vi "Queue_0125.vi"() -> ()   [LabVIEW 2021]
panel:
  out "# elements in queue":i32
  out "Consumer":dbl(graph)
  out "Producer":dbl(graph)
  in  "stop":bool
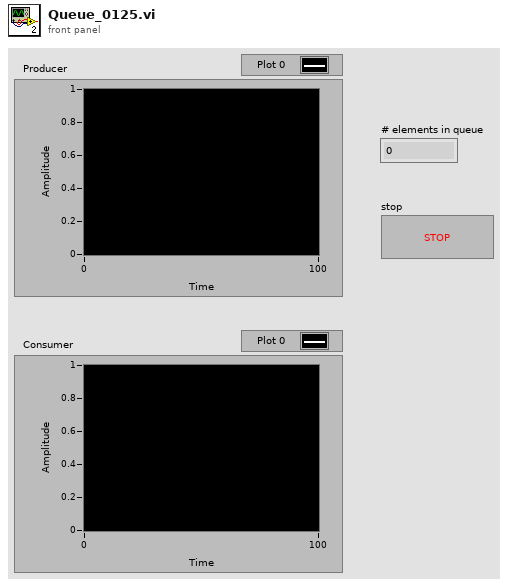
[diagram p1: front panel]
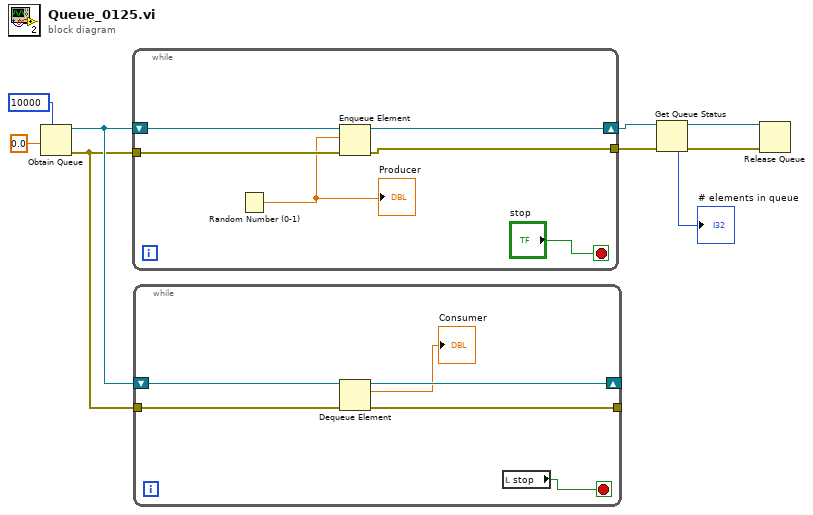
[diagram p0: block diagram]
diagram:
  n1 = Obtain Queue(max queue size (-1, unlimited)=10000, element data type=0.0) -> (queue out=w3:refnum<queue>, error out=w2:errorcluster)  [unwired: 3 in, 1 out]
  n2 = while {
    shift-right: [w14] -> w7
    shift-left: w3 -> [w15]
    tunnel: w2 -> [w13]
    tunnel: [w12] -> w5
    stop <- "stop" stop-if-true
    n3 = Random Number (0-1)() -> (number: 0 to 1=w10:dbl)
    "Producer" <- w10
    n4 = Enqueue Element(queue=w15, element=w10, error in (no error)=w13) -> (queue out=w14:refnum<queue>, error out=w12:errorcluster)  [unwired: 1 in, 1 out]
  }
  n5 = while {
    shift-right: [w20] -> _
    shift-left: w3 -> [w21]
    tunnel: w2 -> [w19]
    tunnel: [w18] -> _
    stop <- w17 stop-if-true
    n6 = Dequeue Element(queue=w21, error in (no error)=w19) -> (queue out=w20:refnum<queue>, element=→"Consumer":dbl, error out=w18:errorcluster)  [unwired: 1 in, 1 out]
    n7 = local read "stop"() -> (w17:bool)
  }
  n8 = Get Queue Status(queue=w7, error in (no error)=w5) -> (queue out=w6:refnum<queue>, error out=w4:errorcluster, # elements in queue=→"# elements in queue":i32)  [unwired: 1 in, 5 out]
  n9 = Release Queue(queue=w6, error in (no error)=w4) -> ()  [unwired: 1 in, 3 out]
